vi "set_FPGA_reference.vi"(8 "error in (no error)":errorcluster, 10 "FPGA VI reference":T1, 11 "FPGAWrapperDL090211Galvo in":refnum<class "FPGAWrapperDL090211Galvo.lvclass">) -> (0 "error out":errorcluster, 3 "FPGAWrapperDL090211Galvo out":refnum<class "FPGAWrapperDL090211Galvo.lvclass">)   [LabVIEW 2010, in "FPGAWrapperDL090211Galvo.lvclass"]
uses:
  FPGAWrapperDL090211Galvo.lvclass
  FPGA_VI_ref.ctl
  class_data.vi
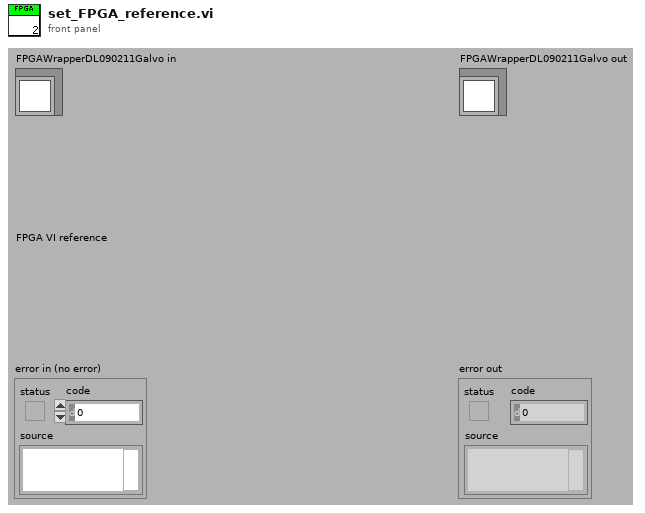
[diagram p1: front panel]
types:
  T1 = typedef "FPGAWrapperDL090211Galvo.lvclass/FPGA_VI_ref.ctl" = refnum<k20>
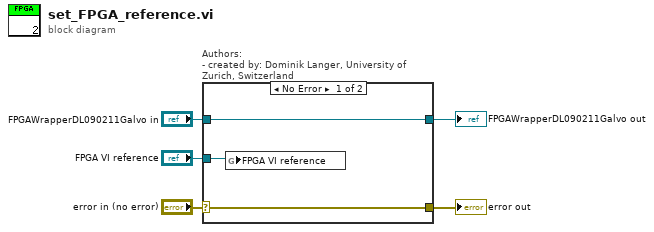
[diagram p0: block diagram]
diagram:
  n1 = case "Authors: \n- created by: Dominik Langer, University of Zurich, Switzerland" shown="No Error" "error in (no error)" {
    selector: "error in (no error)" -> [w7 w10]
    tunnel: [w7 w10] -> w4
    tunnel: [w8 w9] -> w2
    tunnel: "FPGAWrapperDL090211Galvo in" -> [w8 w9]
    tunnel: "FPGA VI reference" -> [w6 _]
    frame No Error {
      n2 = global write "class_data.vi" "FPGA VI reference"(w6) -> ()
    }
    frame Error {
    }
  }
  "error out" <- w4
  "FPGAWrapperDL090211Galvo out" <- w2
